vi "Read.vi"   [LabVIEW 2013, in "Watts Up Series.lvlib"]
doc: "Allows users to read one or more measurements from the DMM."
uses:
  <instrlib>/Watts Up Series/Watts Up Series.lvlib
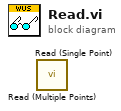
[diagram p0: block diagram]
diagram:
  n1 = call <instrlib>:"Read (Multiple Points).vi"() -> ()  [unwired: 9 in, 3 out]
  n2 = call <instrlib>:"Read (Single Point).vi"() -> ()  [unwired: 9 in, 3 out]
